vi "IR read.vi"(8 "error in (no error)":errorcluster, 11 "IR sensor in":refnum<class "IR sensor.lvclass">) -> (0 "error out":errorcluster, 2 "IR":u16, 3 "IR sensor out":refnum<class "IR sensor.lvclass">)   [LabVIEW 2019, in "my FPGA lib.lvlib" / "IR sensor.lvclass"]
uses:
  IR sensor.lvclass
  IR sensor.lvclass/IR sensor.ctl
  <vilib>/Utility/error.llb/Error Cluster From Error Code.vi
  <vilib>/rvi/errors/niLvFpgaAdjustHostInterfaceError.vi
  <vilib>/rvi/interface/nirviReadWriteControl/nirviReadWriteControl.xnode
  NiFpgaLv.dll
  <vilib>/rvi/interface/Simulation/niFpgaSimulationCallBeginRW.vi
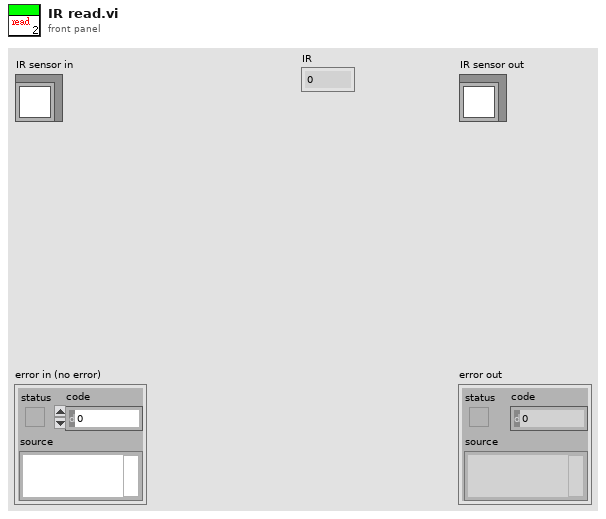
[diagram p1: front panel]
types:
  T1 = enum16{"IR.1", "IR.2", "IR.3", "IR.4", "IR.5", "IR.6", "IR.7", "IR.8"}
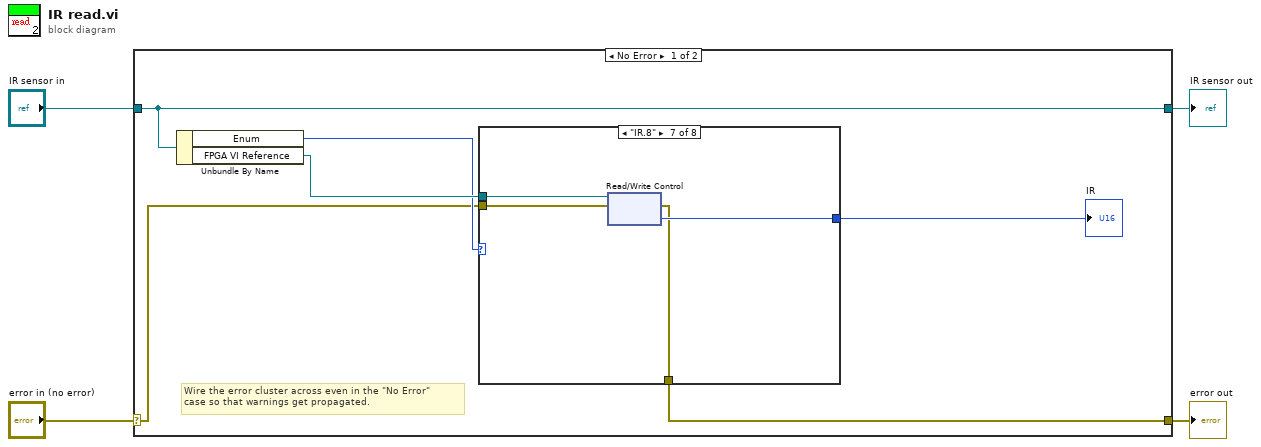
[diagram p0: block diagram]
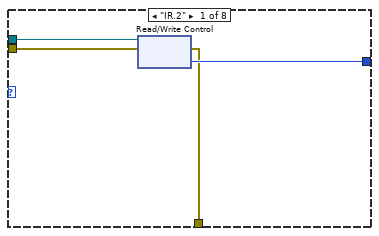
[diagram p2: hidden frame]
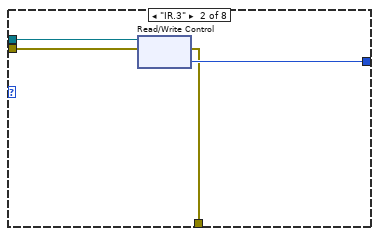
[diagram p3: hidden frame]
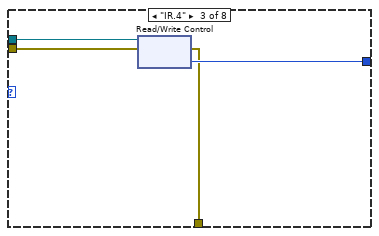
[diagram p4: hidden frame]
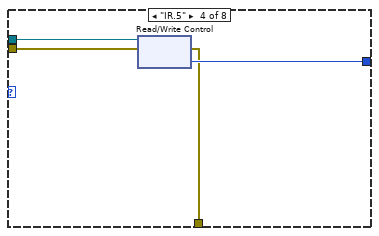
[diagram p5: hidden frame]
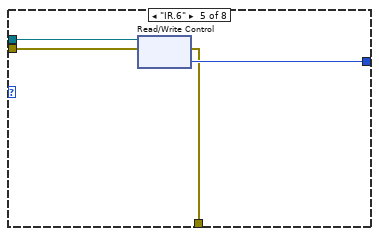
[diagram p6: hidden frame]
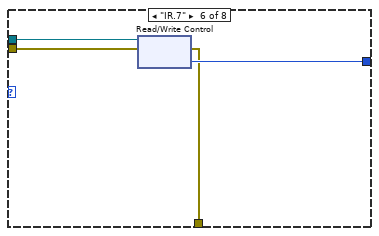
[diagram p7: hidden frame]
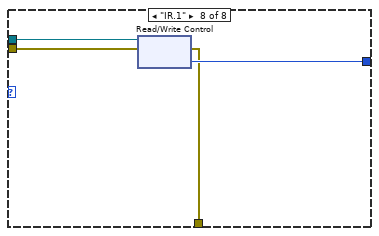
[diagram p8: hidden frame]
diagram:
  n1 = case shown="No Error" "error in (no error)" {
    selector: "error in (no error)" -> [w7 w44]
    tunnel: [w5 w44] -> w3
    tunnel: [w10 w43] -> w1
    tunnel: "IR sensor in" -> [w10 w43]
    frame No Error {
      # "Wire the error cluster across even in the \"No Error\"\ncase so that warnings get propagated."
      n2 = Unbundle By Name(w10) -> ("Enum"=w8:T1, "FPGA VI Reference"=w9:refnum<k20>)
      n3 = case shown="\"IR.8\"" w8 {
        tunnel: w9 -> [w14 w18 w22 w26 w30 w34 w38 w42]
        tunnel: w7 -> [w13 w17 w21 w25 w29 w33 w37 w41]
        tunnel: [w12 w16 w20 w24 w28 w32 w36 w40] -> w6
        tunnel: [w11 w15 w19 w23 w27 w31 w35 w39] -> w5
        frame "IR.2" {
          n4 = xnode "Read/Write Control"("FPGA VI Reference In"=w14, "error in"=w13) -> ("error out"=w11:errorcluster, "IR 2"=w12:u16)  [unwired: 1 out]
        }
        frame "IR.3" {
          n5 = xnode "Read/Write Control"("FPGA VI Reference In"=w18, "error in"=w17) -> ("error out"=w15:errorcluster, "IR 3"=w16:u16)  [unwired: 1 out]
        }
        frame "IR.4" {
          n6 = xnode "Read/Write Control"("FPGA VI Reference In"=w22, "error in"=w21) -> ("error out"=w19:errorcluster, "IR 4"=w20:u16)  [unwired: 1 out]
        }
        frame "IR.5" {
          n7 = xnode "Read/Write Control"("FPGA VI Reference In"=w26, "error in"=w25) -> ("error out"=w23:errorcluster, "IR 5"=w24:u16)  [unwired: 1 out]
        }
        frame "IR.6" {
          n8 = xnode "Read/Write Control"("FPGA VI Reference In"=w30, "error in"=w29) -> ("error out"=w27:errorcluster, "IR 6"=w28:u16)  [unwired: 1 out]
        }
        frame "IR.7" {
          n9 = xnode "Read/Write Control"("FPGA VI Reference In"=w34, "error in"=w33) -> ("error out"=w31:errorcluster, "IR 7"=w32:u16)  [unwired: 1 out]
        }
        frame "IR.8" {
          n10 = xnode "Read/Write Control"("FPGA VI Reference In"=w38, "error in"=w37) -> ("error out"=w35:errorcluster, "IR 8"=w36:u16)  [unwired: 1 out]
        }
        frame "IR.1" {
          n11 = xnode "Read/Write Control"("FPGA VI Reference In"=w42, "error in"=w41) -> ("error out"=w39:errorcluster, "IR 1"=w40:u16)  [unwired: 1 out]
        }
      }
      "IR" <- w6
    }
    frame Error {
    }
  }
  "error out" <- w3
  "IR sensor out" <- w1
